vi "Test Settings API.vi"() -> ()   [LabVIEW 2022 SP3]
doc: "Settings API Tester."
uses:
  Settings.lvlib
  <vilib>/Utility/error.llb/DialogType.ctl
  Libraries/hse-libraries/Source/hse-dqmh/hse-dqmh.lvlib
  <vilib>/Hampel Software Engineering/HSE Logger/hse-logger.lvlib
  <vilib>/Hampel Software Engineering/HSE Logger/LogRecord/LogRecord.lvclass
  Framework/UI Manager/Module Display Scenarios.ctl
  Framework/UI Manager/UI Manager.lvlib
panel:
  in  "Scenario":T1
  in  "Request UI Display":bool
  in  "Configure":bool
  in  "Prepare":bool
  out "last error":errorcluster
  in  "Show Diagram on Init":bool
  in  "wait for reply":bool=TRUE
  in  "Show Block Diagram":bool
  in  "X":dbl=1.0
  out "Reply Payload":dbl
  in  "Stop Module":bool
  in  "Start Module":bool
  out "Do Something Count":i32
  in  "Test Do Something Else and Wait for Reply":bool
  in  "Hide Module Panel":bool
  in  "Show Module Panel":bool
  in  "Test Do Something Else":bool
  in  "Test Do Something":bool
  out "Status":string
  out "Module Running?":bool
  # "This VI tests the API for the Module."
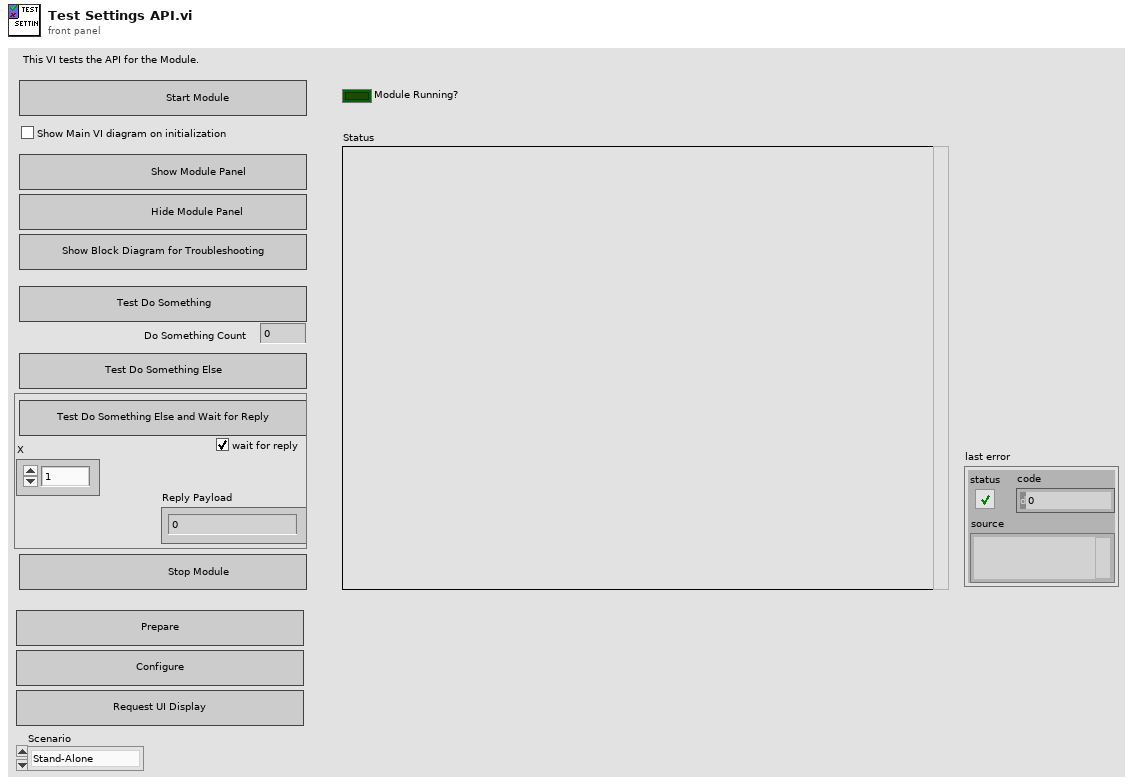
[diagram p1: front panel]
types:
  T1 = typedef "UI Manager.lvlib/Module Display Scenarios.ctl" = enum16{"Stand-Alone", "Managed"}
  T2 = typedef "Settings.lvlib/Broadcast Events--cluster.ctl" = cluster{"Module Did Init":refnum<user-event>, "Status Updated":refnum<user-event>, "Error Reported":refnum<user-event>, "Did Something":refnum<user-event>, "Module Did Stop":refnum<user-event>, "Update Module Execution Status":refnum<user-event>, "System Message":refnum<user-event>}
  T3 = typedef "DialogType.ctl" = u16
  T4 = typedef "Settings.lvlib/Do Something Else and Wait (Reply Payload)--cluster.ctl" = cluster{"Value":dbl, "error":errorcluster}
  T5 = typedef "hse-logger.lvlib/LogLevel.ctl" = enum16{"DEBUG", "INFO", "WARNING", "ERROR", "CRITICAL"}
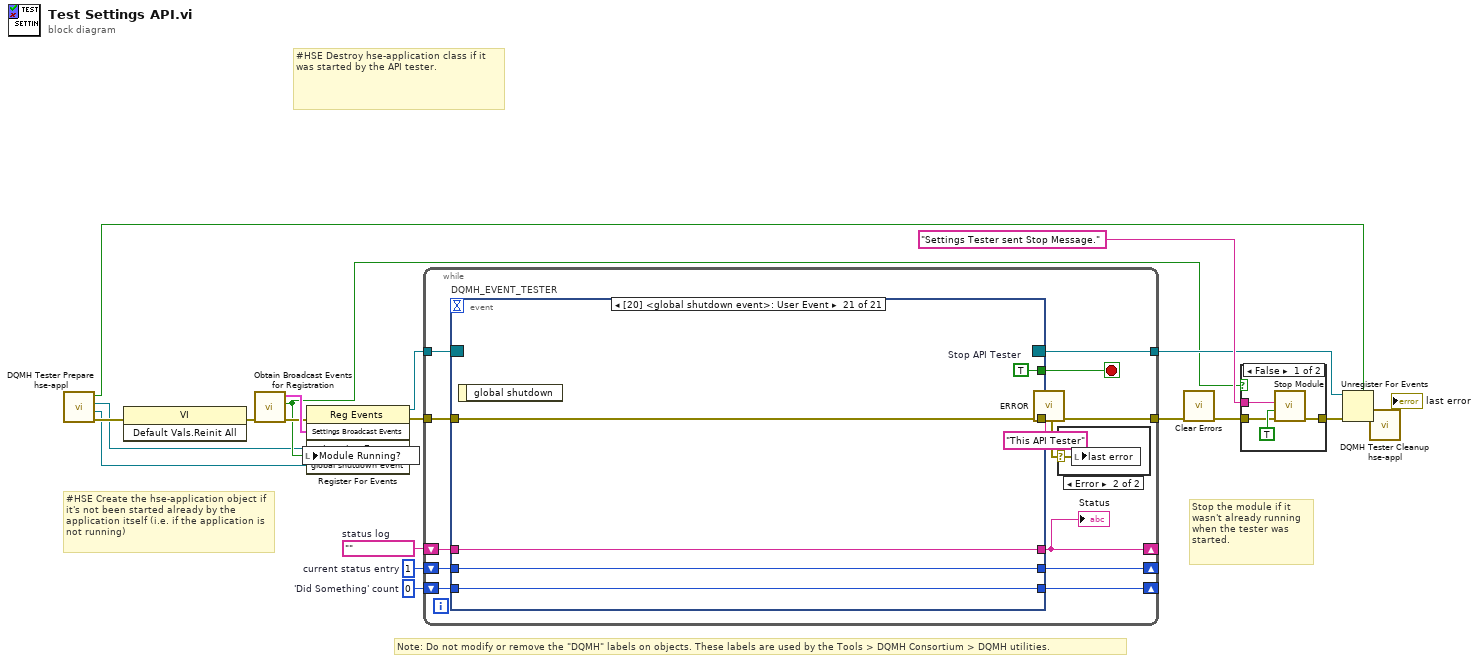
[diagram p0: block diagram]
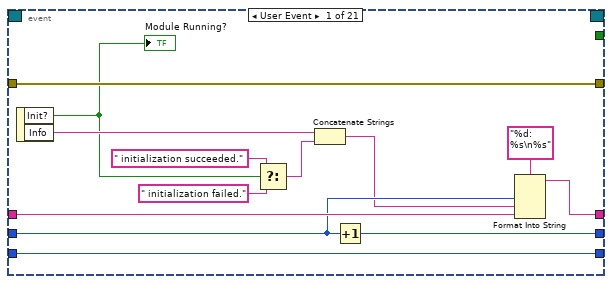
[diagram p4: hidden frame]
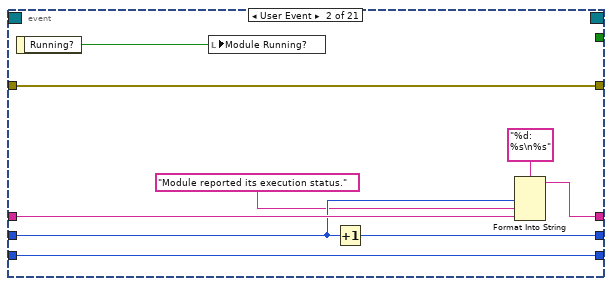
[diagram p5: hidden frame]
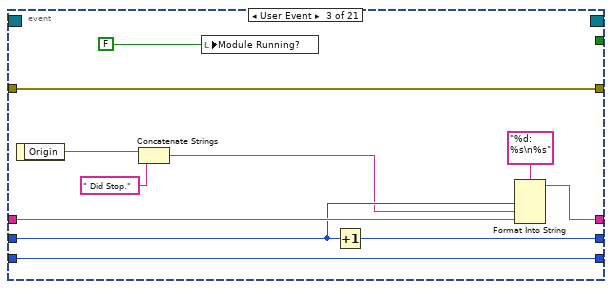
[diagram p6: hidden frame]
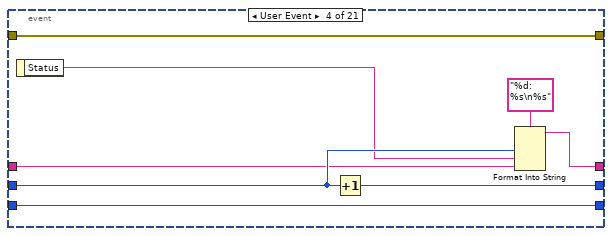
[diagram p7: hidden frame]
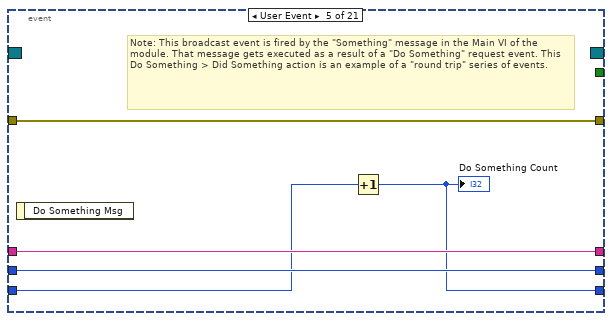
[diagram p8: hidden frame]
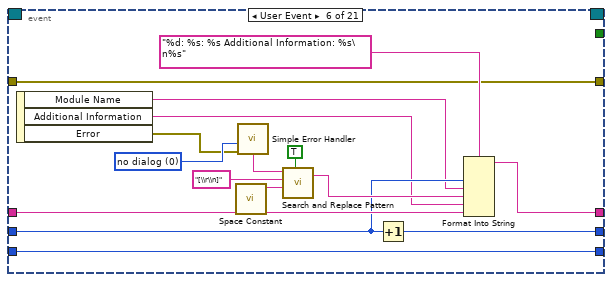
[diagram p9: hidden frame]
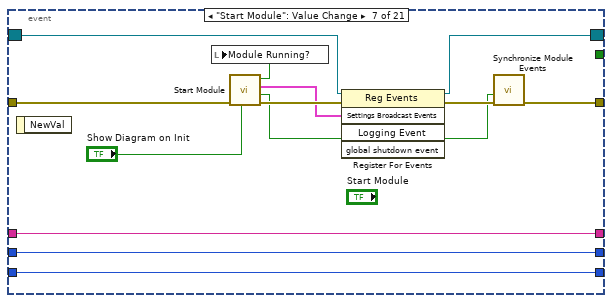
[diagram p10: hidden frame]
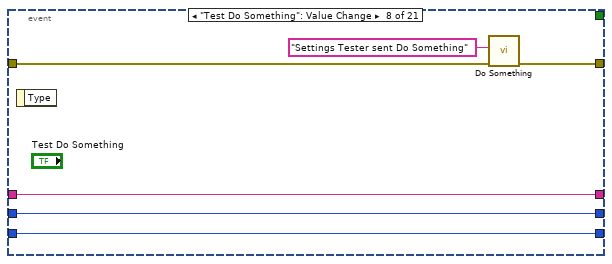
[diagram p11: hidden frame]
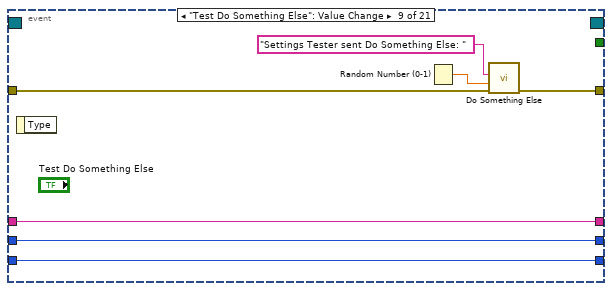
[diagram p12: hidden frame]
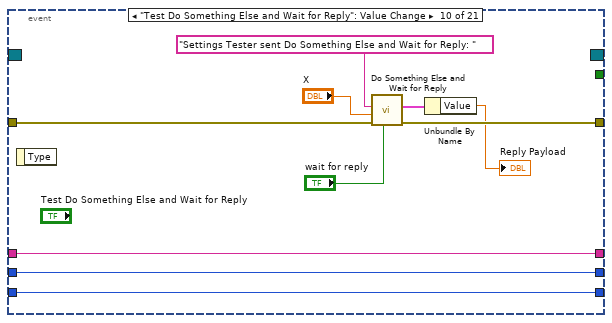
[diagram p13: hidden frame]
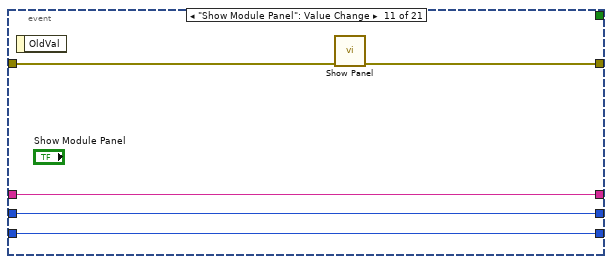
[diagram p14: hidden frame]
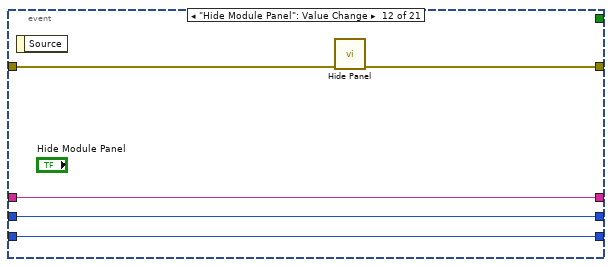
[diagram p15: hidden frame]
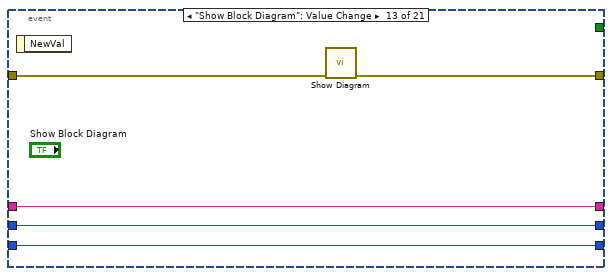
[diagram p16: hidden frame]
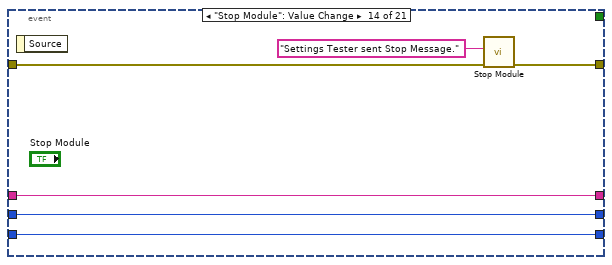
[diagram p17: hidden frame]
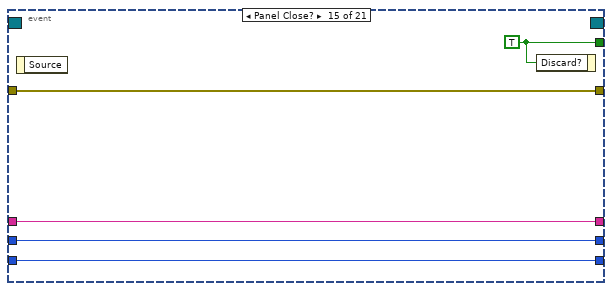
[diagram p18: hidden frame]
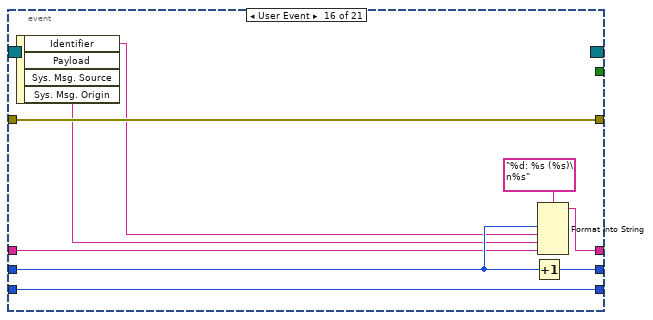
[diagram p19: hidden frame]
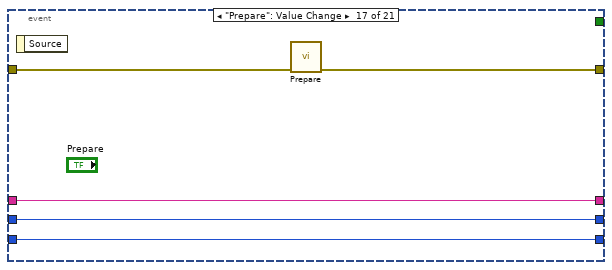
[diagram p20: hidden frame]
diagram:
  w16 = 0  # 'Did Something' count
  w17 = 1  # current status entry
  w18 = ""  # status log
  # "#HSE Destroy hse-application class if it was started by the API tester."
  # "#HSE Create the hse-application object if it's not been started already by the  application itself (i.e. if the application is not running)"
  # "Stop the module if it wasn't already running when the tester was started."
  # "Note: Do not modify or remove the \"DQMH\" labels on objects. These labels are used by the Tools > DQMH Consortium > DQMH utilities."
  n1 = call "DQMH Tester Prepare hse-appl.vi"() -> ("error out"=w6:errorcluster, "global shutdown event"=w5:refnum<user-event>, "Logging Event"=w4:refnum<user-event>, "Started?"=w1:bool)  [unwired: 8 in]
  n2 = invoke class="VI" method="Default Vals.Reinit All"(error in=w6) -> (error out=w11:errorcluster)  [unwired: 2 in, 2 out]
  n3 = call "Obtain Broadcast Events for Registration.vi"("error in"=w11) -> ("error out"=w10:errorcluster, "Already running?"=w9:bool, "Settings Broadcast Events"=w14:T2)  [unwired: 8 in]
  n4 = local write "Module Running?"(w9) -> ()
  n5 = register-events(error in=w10, w14, w4, w5) -> (reference out=w13:refnum<event-registration>, error out=w15:errorcluster)  [unwired: 1 in]
  n6 = while {
    tunnel: w13 -> [w33]
    tunnel: [w23] -> w8
    shift-right: [w29] -> _
    shift-left: w18 -> [w31]
    shift-right: [w30] -> _
    shift-left: w17 -> [w32]
    shift-right: [w27] -> _
    shift-left: w16 -> [w28]
    tunnel: w15 -> [w26]
    tunnel: [w25] -> w12
    stop <- w21 stop-if-true
    n7 = event "DQMH_EVENT_TESTER" shown="[20] <global shutdown event>: User Event" {
      selector: w33 -> [_ _ _ _ _ _ w102 _ _ _ _ _ _ _ _ _ _ _ _ _ _]
      dyn-events: [_ _ _ _ _ _ w101 _ _ _ _ _ _ _ _ _ _ _ _ _ _] -> w25
      timeout: _ -> [_ _ _ _ _ _ _ _ _ _ _ _ _ _ _ _ _ _ _ _ _]
      tunnel: [w47 w49 w57 w68 w76 w84 w100 w115 w122 w132 w137 w142 w143 w150 w154 w167 w168 w173 w179 w202 w209] -> w24
      tunnel: w32 -> [w44 w54 w65 w72 w79 w87 w106 w112 w118 w129 w135 w140 w145 w152 w156 w164 w170 w175 w181 w199 w207]
      tunnel: w31 -> [w45 w55 w66 w71 w80 w88 w107 w113 w119 w130 w136 w141 w146 w153 w157 w161 w171 w176 w182 w198 w208]
      tunnel: [w42 w52 w63 w73 w80 w86 w107 w113 w119 w130 w136 w141 w146 w153 w157 w165 w171 w176 w182 w200 w208] -> w29
      tunnel: [w43 w53 w64 w75 w79 w85 w106 w112 w118 w129 w135 w140 w145 w152 w156 w163 w170 w175 w181 w201 w207] -> w30
      tunnel: w28 -> [w39 w50 w59 w69 w78 w96 w105 w111 w117 w128 w134 w139 w144 w151 w155 w166 w169 w174 w180 w203 w206]
      tunnel: [w39 w50 w59 w69 w77 w96 w105 w111 w117 w128 w134 w139 w144 w151 w155 w166 w169 w174 w180 w203 w206] -> w27
      tunnel: w26 -> [w47 w49 w57 w68 w76 w84 w99 w110 w116 w125 w133 w138 w147 w148 w154 w167 w172 w177 w183 w204 w209]
      tunnel: [_ _ _ _ _ _ _ _ _ _ _ _ _ _ w158 _ _ _ _ _ w205] -> w21
      event User Event {
        n8 = event-data() -> ("Init?"=w38:bool, "Info"=w41:string)  [unwired: 1 in]
        "Module Running?" <- w38
        n9 = Select(t=" initialization succeeded.", s=w38, f=" initialization failed.") -> (s? t:f=w35:string)
        n10 = Concatenate Strings(w41, w35) -> (w40:string)
        n11 = Increment(x=w44) -> (x+1=w43:i32)
        n12 = Format Into String(format string="%d: %s\n%s", w44, w40, w45) -> (resulting string=w42:string)  [unwired: 2 in, 1 out]
      }
      event User Event {
        n13 = event-data() -> ("Running?"=w48:bool)  [unwired: 1 in]
        n14 = local write "Module Running?"(w48) -> ()
        n15 = Increment(x=w54) -> (x+1=w53:i32)
        n16 = Format Into String(format string="%d: %s\n%s", w54, "Module reported its execution status.", w55) -> (resulting string=w52:string)  [unwired: 2 in, 1 out]
      }
      event User Event {
        n17 = event-data() -> ("Origin"=w62:string)  [unwired: 1 in]
        n18 = Concatenate Strings(w62, " Did Stop.") -> (w61:string)
        n19 = local write "Module Running?"(FALSE ("Module Did Init?")) -> ()
        n20 = Increment(x=w65) -> (x+1=w64:i32)
        n21 = Format Into String(format string="%d: %s\n%s", w65, w61, w66) -> (resulting string=w63:string)  [unwired: 2 in, 1 out]
      }
      event User Event {
        n22 = event-data() -> ("Status"=w70:string)  [unwired: 1 in]
        n23 = Increment(x=w72) -> (x+1=w75:i32)
        n24 = Format Into String(format string="%d: %s\n%s", w72, w70, w71) -> (resulting string=w73:string)  [unwired: 2 in, 1 out]
      }
      event User Event {
        # "Note: This broadcast event is fired by the \"Something\" message in the Main VI of the module. That message gets executed as a result of a \"Do Something\" request event. This Do Something > Did Something action is an example of a \"round trip\" series of events."
        n25 = event-data() -> ()  [unwired: 1 in, 1 out]
        n26 = Increment(x=w78) -> (x+1=w77:i32)
        "Do Something Count" <- w77
      }
      event User Event {
        w89 = T3 0 items=["no dialog", "OK message", "continue or stop message", "OK message + warnings", "continue/stop + warnings"] ("type of dialog (OK msg:1)")
        n27 = event-data() -> ("Module Name"=w83:string, "Additional Information"=w82:string, "Error"=w81:errorcluster)  [unwired: 1 in]
        n28 = call <vilib>:"Space Constant.vi"() -> ("String"=w93:string)
        n29 = call <vilib>:"Simple Error Handler.vi"("type of dialog (OK msg:1)"=w89, "error in (no error)"=w81) -> ("message"=w90:string)  [unwired: 3 in, 4 out]
        n30 = call <vilib>:"Search and Replace Pattern.vi"("string"=w90, "regular expression (\"\")"="[\\r\\n]" ("regular expression (\"\")"), "replace string (\"\")"=w93, "replace all? (F)"=TRUE ("replace all CR/LF with spaces")) -> ("result string"=w91:string)  [unwired: 1 in, 1 out]
        n31 = Increment(x=w87) -> (x+1=w85:i32)
        n32 = Format Into String(format string="%d: %s: %s Additional Information: %s\n%s", w87, w83, w91, w82, w88) -> (resulting string=w86:string)  [unwired: 2 in, 1 out]
      }
      event "Start Module": Value Change {
        n33 = event-data() -> ()  [unwired: 1 in, 1 out]
        n34 = call "Start Module.vi"("Show Main VI Diagram on Init (F)"="Show Diagram on Init", "error in"=w99) -> ("error out"=w108:errorcluster, "Wait for Event Sync?"=w104:bool, "Settings Broadcast Events"=w103:T2, "Module Was Already Running?"=w98:bool)  [unwired: 6 in]
        n35 = local write "Module Running?"(w98) -> ()
        n36 = register-events(reference=w102, error in=w108, w103) -> (reference out=w101:refnum<event-registration>, error out=w109:errorcluster)  [unwired: 2 in]
        n37 = call "Synchronize Module Events.vi"("error in"=w109, "Wait for Event Sync?"=w104) -> ("error out"=w100:errorcluster)  [unwired: 9 in]
      }
      event "Test Do Something": Value Change {
        n38 = event-data() -> ()  [unwired: 1 in, 1 out]
        n39 = call "Do Something.vi"("error in"=w110, "Do Something Message"="Settings Tester sent Do Something") -> ("error out"=w115:errorcluster)  [unwired: 9 in]
      }
      event "Test Do Something Else": Value Change {
        n40 = event-data() -> ()  [unwired: 1 in, 1 out]
        n41 = Random Number (0-1)() -> (number: 0 to 1=w120:dbl)
        n42 = call "Do Something Else.vi"("error in"=w116, "X"=w120, "Do Something Else Message"="Settings Tester sent Do Something Else: " ("Do Something Message")) -> ("error out"=w122:errorcluster)  [unwired: 8 in]
      }
      event "Test Do Something Else and Wait for Reply": Value Change {
        n43 = event-data() -> ()  [unwired: 1 in, 1 out]
        n44 = call "Do Something Else and Wait for Reply.vi"("wait for reply (T)"="wait for reply", "error in"=w125, "X"="X", "Do Something Else Message"="Settings Tester sent Do Something Else and Wait for Reply: " ("Do Something Message")) -> ("error out"=w132:errorcluster, "Reply Payload"=w127:T4)  [unwired: 5 in, 1 out]
        n45 = Unbundle By Name(w127) -> ("Value"=→"Reply Payload":dbl)
      }
      event "Show Module Panel": Value Change {
        n46 = event-data() -> ()  [unwired: 1 in, 1 out]
        n47 = call "Show Panel.vi"("error in"=w133) -> ("error out"=w137:errorcluster)  [unwired: 10 in]
      }
      event "Hide Module Panel": Value Change {
        n48 = event-data() -> ()  [unwired: 1 in, 1 out]
        n49 = call "Hide Panel.vi"("error in"=w138) -> ("error out"=w142:errorcluster)  [unwired: 10 in]
      }
      event "Show Block Diagram": Value Change {
        n50 = event-data() -> ()  [unwired: 1 in, 1 out]
        n51 = call "Show Diagram.vi"("error in"=w147) -> ("error out"=w143:errorcluster)  [unwired: 10 in]
      }
      event "Stop Module": Value Change {
        n52 = event-data() -> ()  [unwired: 1 in, 1 out]
        n53 = call "Stop Module.vi"("error in"=w148, "Origin"="Settings Tester sent Stop Message.") -> ("error out"=w150:errorcluster)  [unwired: 9 in]
      }
      event Panel Close? {
        w158 = TRUE ("Discard?")
        n54 = event-data() -> ()  [unwired: 1 in, 1 out]
        n55 = event-data("Discard?"=w158) -> ()  [unwired: 1 in, 1 out]
      }
      event User Event {
        n56 = event-data() -> ("Identifier"=w160:string, "Sys. Msg. Origin"=w159:string)  [unwired: 1 in, 2 out]
        n57 = Increment(x=w164) -> (x+1=w163:i32)
        n58 = Format Into String(format string="%d: %s (%s)\n%s", w164, w160, w159, w161) -> (resulting string=w165:string)  [unwired: 2 in, 1 out]
      }
      event "Prepare": Value Change {
        n59 = event-data() -> ()  [unwired: 1 in, 1 out]
        n60 = call "Prepare.vi"("error in"=w172) -> ("error out"=w168:errorcluster)  [unwired: 10 in]
      }
      event "Configure": Value Change {
        n61 = event-data() -> ()  [unwired: 1 in, 1 out]
        n62 = call "Configure.vi"("error in"=w177) -> ("error out"=w173:errorcluster)  [unwired: 10 in]
      }
      event "Request UI Display": Value Change {
        n63 = event-data() -> ()  [unwired: 1 in, 1 out]
        n64 = call "Request UI Display.vi"("error in"=w183, "Scenario"="Scenario") -> ("error out"=w179:errorcluster)  [unwired: 8 in, 1 out]
      }
      event User Event {
        n65 = event-data() -> ("LogRecord"=w197:refnum<class "LogRecord.lvclass">)  [unwired: 1 in]
        n66 = call <vilib>:"Get ISO Time.vi"("error in"=w204, "LogRecord in"=w197) -> ("error out"=w189:errorcluster, "ISO Time"=w191:string, "LogRecord out"=w184:refnum<class "LogRecord.lvclass">)  [unwired: 7 in]
        n67 = call <vilib>:"Get Level.vi"("error in"=w189, "LogRecord in"=w184) -> ("error out"=w188:errorcluster, "Level"=w192:T5, "LogRecord out"=w185:refnum<class "LogRecord.lvclass">)  [unwired: 7 in]
        n68 = call <vilib>:"Get Message.vi"("error in"=w188, "LogRecord in"=w185) -> ("error out"=w187:errorcluster, "Message"=w193:string, "LogRecord out"=w186:refnum<class "LogRecord.lvclass">)  [unwired: 7 in]
        n69 = call <vilib>:"Get Error.vi"("error in"=w187, "LogRecord in"=w186) -> ("error out"=w202:errorcluster, "Error"=w194:errorcluster)  [unwired: 7 in, 1 out]
        n70 = Unbundle By Name(w194) -> ("code"=w195:i32, "source"=w196:string)
        n71 = Format Into String(format string="%d: HSE-Logger: %s - %s - %s - %d: %s\n%s", w199, w191, w192, w193, w195, w196, w198) -> (resulting string=w200:string)  [unwired: 2 in, 1 out]
        n72 = Increment(x=w199) -> (x+1=w201:i32)
      }
      event User Event {
        w205 = TRUE  # Stop API Tester
        n73 = event-data() -> ()  [unwired: 1 in, 1 out]
      }
    }
    "Status" <- w29
    n74 = call <vilib>:"ERROR.vi"("Message"="This API Tester", "error in"=w24) -> ("error out"=w23:errorcluster)  [unwired: 9 in]
    n75 = case shown="Error" w23 {
      selector: w23 -> [_ w34]
      frame No Error {
      }
      frame Error {
        n76 = local write "last error"(w34) -> ()
      }
    }
  }
  n77 = call <vilib>:"Clear Errors.vi"("error in (no error)"=w8) -> ("error out"=w3:errorcluster)  [unwired: 5 in, 1 out]
  n78 = case shown="False" w9 {
    tunnel: [w213 w214] -> w20
    tunnel: "Settings Tester sent Stop Message." ("Origin") -> [w212 _]
    tunnel: w3 -> [w210 w214]
    frame False {
      n79 = call "Stop Module.vi"("error in"=w210, "Wait for Module to Stop? (F)"=TRUE ("Wait for Module to stop?"), "Origin"=w212) -> ("error out"=w213:errorcluster)  [unwired: 8 in]
    }
    frame True {
    }
  }
  n80 = Unregister For Events(event registration refnum=w12, error in=w20) -> (error out=w7:errorcluster)
  n81 = call "DQMH Tester Cleanup hse-appl.vi"("error in"=w7, "Stop?"=w1) -> ("error out"=→"last error":errorcluster)  [unwired: 9 in]
